vi "MCListbox Refresh.vi"(6 "Which Cells":T1(ring), 8 "Error In":errorcluster, 9 "color of New Cells":u32(colorbox)=16777225, 10 "color of Blank cells":u32(colorbox)=16777238, 11 "MulticolumnListbox in":refnum<vi>) -> (0 "Error Out":errorcluster, 3 "MulticolumnListbox out":refnum<vi>)   [LabVIEW 2013]
uses:
  <vilib>/Utility/miscctls.llb/LVRowAndColumnTypeDef.ctl
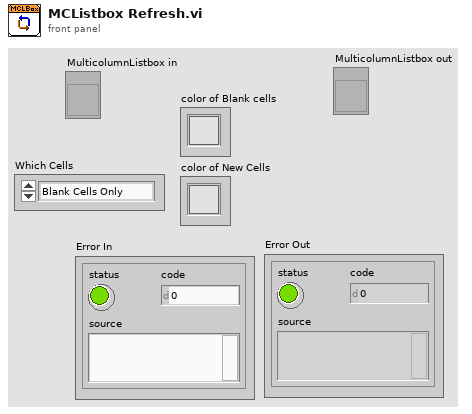
[diagram p1: front panel]
types:
  T1 = enum16{"Blank Cells Only", "Exisiting and Blank Cells"}
  T2 = typedef "LVRowAndColumnTypeDef.ctl" = cluster{"Row":i32, "Column":i32}
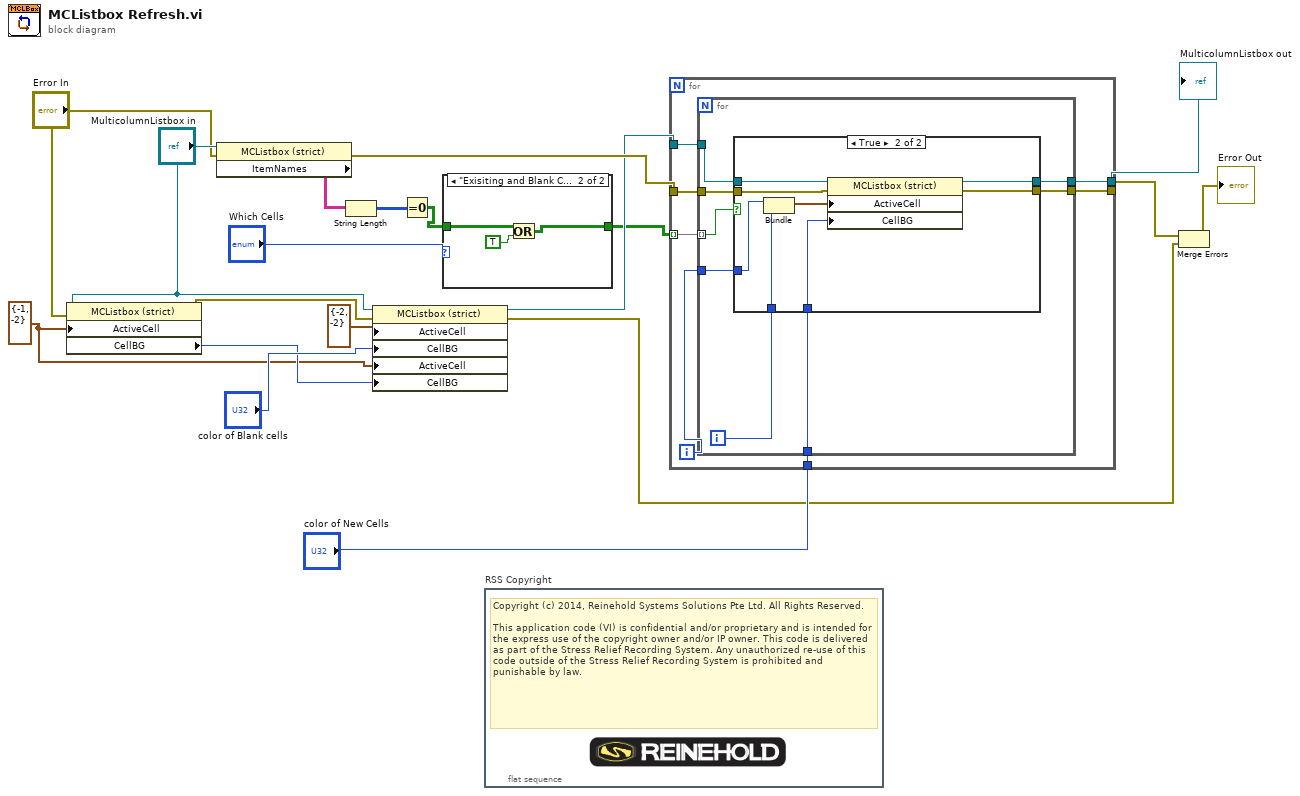
[diagram p0: block diagram]
diagram:
  w16 = T2 {"Row"=-1, "Column"=-2} ("Active Cell:Active Cell")
  n1 = property on="Property Node" class="MCListbox (strict)"(reference="MulticolumnListbox in", error in="Error In", "ActiveCell"=w16) -> (error out=w18:errorcluster, "CellBG"=w17:u32)  [unwired: 1 out]
  n2 = property on="Property Node" class="MCListbox (strict)"(reference="MulticolumnListbox in", error in="Error In") -> (error out=w10:errorcluster, "ItemNames"=w7:string[][])  [unwired: 1 out]
  n3 = String Length(string=w7) -> (length=w13:i32[][])
  n4 = property on="Property Node" class="MCListbox (strict)"(reference="MulticolumnListbox in", error in=w18, "ActiveCell"=T2 {"Row"=-2, "Column"=-2} ("Active Cell:Active Cell"), "CellBG"="color of Blank cells", "ActiveCell"=w16, "CellBG"=w17) -> (reference out=w9:refnum<vi>, error out=w2:errorcluster)
  n5 = Equal To 0?(x=w13) -> (x = 0?=w5:bool[][])
  n6 = case shown="\"Exisiting and Blank Cells\"" "Which Cells" {
    tunnel: w5 -> [w20 w23]
    tunnel: [w20 w21] -> w4
    frame "Blank Cells Only", Default {
    }
    frame "Exisiting and Blank Cells" {
      n7 = Or(x=w23, y=TRUE) -> (x .or. y?=w21:bool[][])
    }
  }
  n8 = flat-sequence "RSS Copyright" {
    frame #0 {
      # "Copyright (c) 2014, Reinehold Systems Solutions Pte Ltd. All Rights Reserved.\n\nThis application code (VI) is confidential and/or proprietary and is intended for the express use of the copyright owner and/or IP owner. This code is delivered as part of the Stress Relief Recording System. Any unauthorized re-use of this code outside of the Stress Relief Recording System is prohibited and punishable by law."
    }
  }
  n9 = for {
    tunnel: w4 -> [w30] mode=indexing
    tunnel: "color of New Cells" -> [w28]
    tunnel: w9 -> [w27]
    tunnel: [w26] -> w3
    tunnel: w10 -> [w25]
    tunnel: [w24] -> w8
    i -> [w29]
    n10 = for {
      tunnel: w30 -> [w38] mode=indexing
      tunnel: w29 -> [w37]
      tunnel: w28 -> [w35]
      tunnel: w27 -> [w34]
      tunnel: [w33] -> w26
      tunnel: w25 -> [w32]
      tunnel: [w31] -> w24
      i -> [w36]
      n11 = case shown="True" w38 {
        tunnel: w37 -> [_ w45]
        tunnel: w36 -> [_ w44]
        tunnel: w35 -> [_ w46]
        tunnel: w34 -> [w39 w43]
        tunnel: [_ w42] -> w33
        tunnel: w32 -> [_ w41]
        tunnel: [w39 w40] -> w31
        frame False {
        }
        frame True {
          n12 = Bundle(w45, w44) -> (w47:cluster{i32, i32})  [unwired: 1 in]
          n13 = property on="Property Node" class="MCListbox (strict)"(reference=w43, error in=w41, "ActiveCell"=w47, "CellBG"=w46) -> (reference out=w40:refnum<vi>, error out=w42:errorcluster)
        }
      }
    }
  }
  "MulticolumnListbox out" <- w8
  n14 = Merge Errors(w3, w2) -> (→"Error Out":errorcluster)
